vi "Duplicate.vi"(8 "error in":errorcluster, 10 "parameters":variant, 11 "Scope Channel":refnum<class "Scope Channel.lvclass">) -> (0 "error out":errorcluster, 3 "Scope Channel out":refnum<class "Scope Channel.lvclass">)   [LabVIEW 2025, in "Scope.lvlib" / "Scope Channel.lvclass"]
doc: "Implements the specific behavior of a node when it is being duplicated\nCan be used to change the name of the new node for example adding Copy to it. \nCopyright 2017 National Instruments Corporation\n\nLicensed under the Apache License, Version 2.0 (the \"License\"); you may not use this file except in compliance with the License. You may obtain a copy of the License at http://www.apache.org/licenses/LICENSE-2.0\nUnless required by applicable law or agreed to in writing, software distributed under the License is distributed on an \"AS IS\" BASIS, WITHOUT WARRANTIES OR CONDITIONS OF ANY KIND, either express or implied. See the License for the specific language governing permissions and limitations under the License."
uses:
  Scope Channel.lvclass
  Scope Channel.lvclass/Scope Channel.ctl
  Scope Channel configuration/Scope Channel configuration.lvclass
  C:/Users/Public/Documents/Sandia National Labs/TSS Plugin/Abstract Engine.lvlibp/Plugin/Abstract/Channel configuration/Channel configuration.lvclass
  Users/Public/Documents/Sandia National Labs/TSS Plugin/Abstract Engine.lvlibp/Plugin/Abstract/Channel configuration/Read Channel Setting.vi
  Users/Public/Documents/Sandia National Labs/TSS Plugin/Abstract Engine.lvlibp/Plugin/Abstract/Channel configuration/Write Channel Setting.vi
  Users/Public/Documents/Sandia National Labs/TSS Plugin/Abstract Engine.lvlibp/Plugin/Abstract/Abstract Channel/Abstract Channel.lvclass
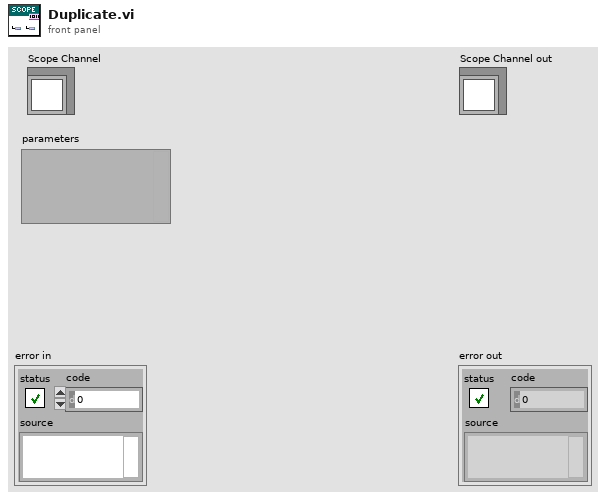
[diagram p1: front panel]
types:
  T1 = typedef "Abstract Engine.lvlibp/Channel configuration.lvclass/Default Channel.ctl" = cluster{"Address":string, "SW Alias":string, "Enabled":bool, "Type":string, "Description":string}
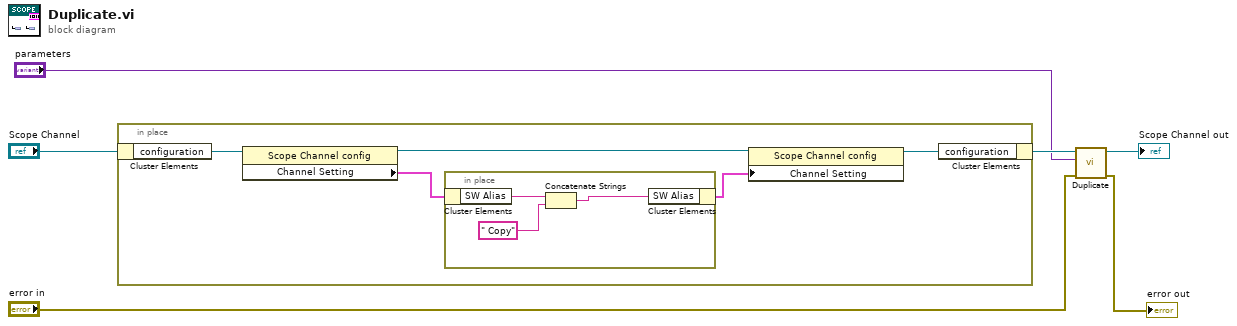
[diagram p0: block diagram]
diagram:
  n1 = in-place {
    n2 = in-place-cluster #1("Scope Channel") -> ("configuration"=w11:refnum<class "Scope Channel configuration.lvclass">)
    n3 = property class="Scope Channel config"(reference=w11) -> (reference out=w9:refnum<class "Scope Channel configuration.lvclass">, "Channel Setting"=w8:T1)  [unwired: 1 in, 1 out]
    n4 = in-place {
      n5 = in-place-cluster #2(w8) -> ("SW Alias"=w14:string)
      n6 = Concatenate Strings(w14, " Copy") -> (w13:string)
      n7 = in-place-cluster #2("SW Alias"=w13) -> (w7:T1)
    }
    n8 = property class="Scope Channel config"(reference=w9, "Channel Setting"=w7) -> (reference out=w10:refnum<class "Scope Channel configuration.lvclass">)  [unwired: 1 in, 1 out]
    n9 = in-place-cluster #1("configuration"=w10) -> (w6:refnum<class "Scope Channel.lvclass">)
  }
  n10 = call-parent "Duplicate.vi"("error in"="error in", "parameters"="parameters", "CEF_Serialize node in"=w6) -> ("error out"=→"error out":errorcluster, "CEF_Serialize node out"=→"Scope Channel out":refnum<class "Scope Channel.lvclass">)  [unwired: 7 in]
